vi "get_S3_by_name.vi"(8 "error in (no error)":errorcluster, 10 "name":string, 11 "MotorSystem in":refnum<class "MotorSystem.lvclass">) -> (0 "error out":errorcluster, 2 "S3":bool, 3 "MotorSystem out":refnum<class "MotorSystem.lvclass">)   [LabVIEW 2016, in "MotionControl_UFO_3DOF.lvlib" / "MotorSystem.lvclass"]
uses:
  <userlib>/MotionControl_UFO_3DOF/MotorSystem/MotorSystem.lvclass
  <userlib>/MotionControl_UFO_3DOF/MotorSystem/MotorSystem.lvclass/MotorSystem.ctl
  <userlib>/MotionControl_UFO_3DOF/OneMotion/OneMotion.lvclass/OneMotion.ctl
  <userlib>/MotionControl_UFO_3DOF/OneMotion/OneMotion.lvclass
  <userlib>/MotionControl_UFO_3DOF/StepMotor/StepMotor.lvclass
  <userlib>/UISimCanFunc_wrapper/UISimCanFunc_wrapper.lvlib
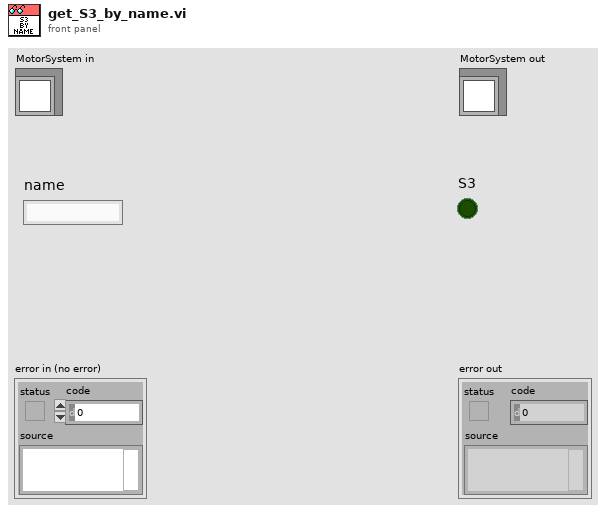
[diagram p1: front panel]
types:
  T1 = typedef "MotionControl_UFO_3DOF.lvlib/MotorSystem.lvclass/MotionCluster.ctl" = cluster{"OneMotion.lvclass":refnum<class "OneMotion.lvclass">, "connected?":bool, "default enabled?":bool, "enabled?":bool}
  T2 = typedef "UISimCanFunc_wrapper.lvlib/SFBK_INFO_OBJ.ctl" = cluster{"bSensor1":bool, "bSensor2":bool, "bSensor3":bool, "fAnaInput":sgl}
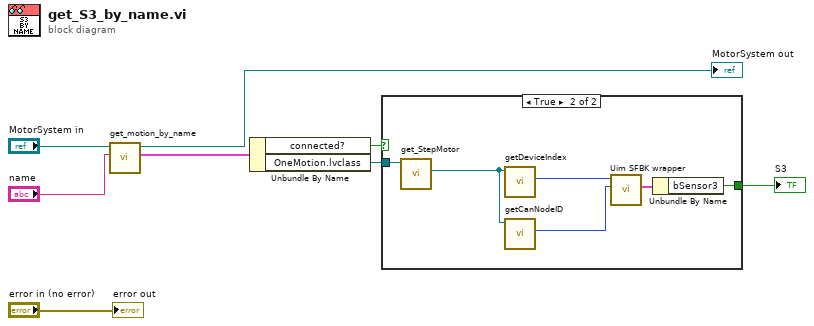
[diagram p0: block diagram]
diagram:
  n1 = call <userlib>:"get_motion_by_name.vi"("name"="name", "MotorSystem in"="MotorSystem in") -> ("motion cluster"=w4:T1, "MotorSystem out"=→"MotorSystem out":refnum<class "MotorSystem.lvclass">)  [unwired: 7 in, 1 out]
  n2 = Unbundle By Name(w4) -> ("connected?"=w1:bool, "OneMotion.lvclass"=w3:refnum<class "OneMotion.lvclass">)
  n3 = case shown="True" w1 {
    tunnel: [_ w10] -> w7
    tunnel: w3 -> [_ w9]
    frame False {
    }
    frame True {
      n4 = call <userlib>:"get_StepMotor.vi"("OneMotion输入"=w9) -> ("StepMotor.lvclass"=w14:refnum<class "StepMotor.lvclass">)  [unwired: 8 in, 2 out]
      n5 = call-dynamic "getDeviceIndex.vi"("StepMotor输入"=w14) -> ("device index"=w13:u32)  [unwired: 8 in, 2 out]
      n6 = call-dynamic "getCanNodeID.vi"("StepMotor输入"=w14) -> ("CAN node ID"=w12:u32)  [unwired: 8 in, 2 out]
      n7 = call <userlib>:"Uim SFBK wrapper.vi"("dwCanNodeId"=w12, "dwDevIndex"=w13) -> ("SFBK_INFO_OBJ"=w11:T2)  [unwired: 7 in, 2 out]
      n8 = Unbundle By Name(w11) -> ("bSensor3"=w10:bool)
    }
  }
  "S3" <- w7
  "error out" <- "error in (no error)"
